vi "Read Applied Torque.vi"(8 "error in (no error)":errorcluster, 10 "Motor ID (0)":u8, 11 "Dynamixel Motor VISA in":refnum<class "Dynamixel Motor VISA.lvclass">) -> (0 "error out":errorcluster, 2 "Load/torque %":sgl, 3 "Dynamixel Motor VISA out":refnum<class "Dynamixel Motor VISA.lvclass">)   [LabVIEW 2016, in "Dynamixel Motor VISA.lvclass"]
doc: "Retrieves the value for the amound of torque the motor is applying."
uses:
  <instrlib>/Dynamixel Motor/HAIOL/VISA/Dynamixel Motor VISA.lvclass
  <instrlib>/Dynamixel Motor/HAIOL/VISA/Dynamixel Motor VISA.lvclass/Dynamixel Motor VISA.ctl
  <instrlib>/Dynamixel Motor/Dynamixel Motor.lvlib
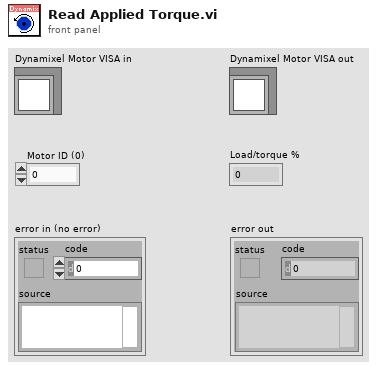
[diagram p1: front panel]
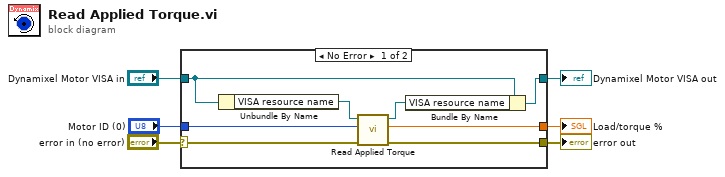
[diagram p0: block diagram]
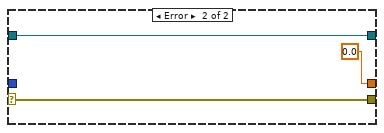
[diagram p2: hidden frame]
diagram:
  n1 = case shown="No Error" "error in (no error)" {
    selector: "error in (no error)" -> [w14 w16]
    tunnel: "Dynamixel Motor VISA in" -> [w9 w17]
    tunnel: "Motor ID (0)" -> [w12 _]
    tunnel: [w11 w16] -> w3
    tunnel: [w10 sgl 0.0 ("Load/torque %")] -> w2
    tunnel: [w7 w17] -> w1
    frame No Error {
      n2 = Unbundle By Name(w9) -> ("VISA resource name"=w13:refnum<visa-resource-name>)
      n3 = call <instrlib>:"Read Applied Torque.vi"("error in (no error)"=w14, "Motor ID (0)"=w12, "VISA resource name"=w13) -> ("error out"=w11:errorcluster, "Load/torque %"=w10:sgl, "VISA resource name out"=w8:refnum<visa-resource-name>)  [unwired: 6 in]
      n4 = Bundle By Name(cluster=w9, "VISA resource name"=w8) -> (w7:refnum<class "Dynamixel Motor VISA.lvclass">)
    }
    frame Error {
    }
  }
  "error out" <- w3
  "Dynamixel Motor VISA out" <- w1
  "Load/torque %" <- w2
